vi "set_safe_mode.vi"(8 "error in (no error)":errorcluster, 10 "exit safe mode? (F)":bool, 11 "LightSourceMH110124MaiTai in":refnum<class "LightSourceMH110124MaiTai.lvclass">) -> (0 "error out":errorcluster, 3 "LightSourceMH110124MaiTai out":refnum<class "LightSourceMH110124MaiTai.lvclass">)   [LabVIEW 2010, in "LightSourceMH110124MaiTai.lvclass"]
uses:
  LightSourceMH110124MaiTai.lvclass
  LightSourceMH110124MaiTai.lvclass/LightSourceMH110124MaiTai.ctl
  class_data.vi
panel:
  out "finished?":bool
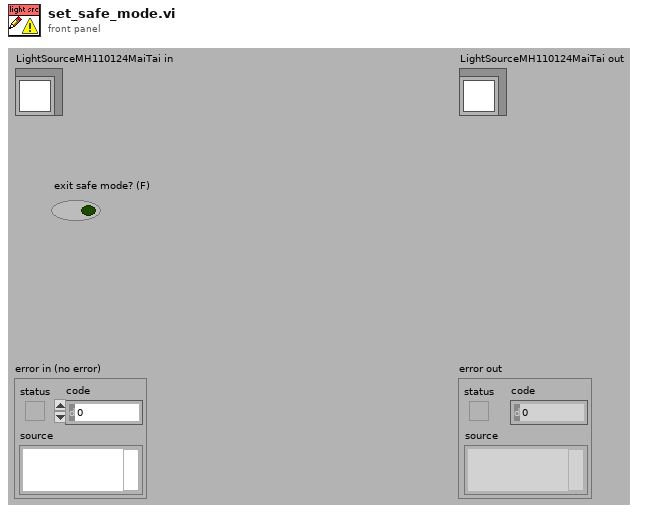
[diagram p1: front panel]
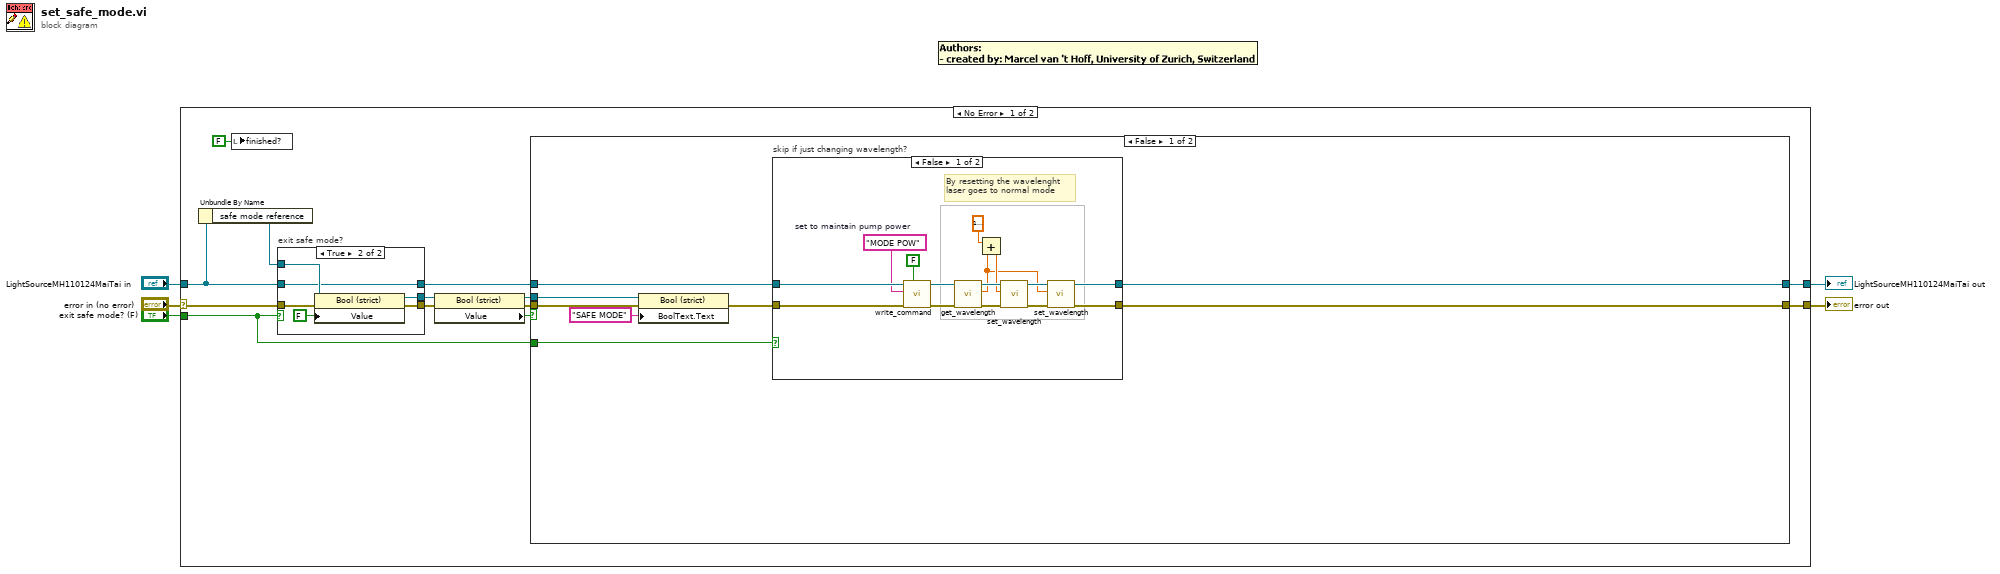
[diagram p0: block diagram]
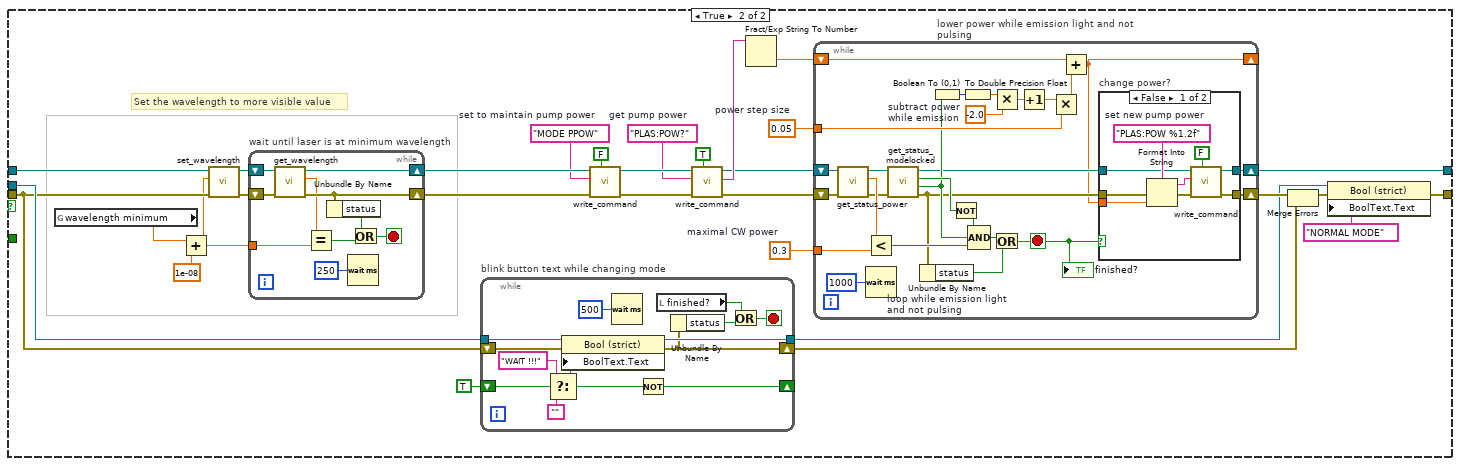
[diagram p4: hidden frame]
diagram:
  n1 = case shown="No Error" "error in (no error)" {
    selector: "error in (no error)" -> [w11 w145]
    tunnel: "LightSourceMH110124MaiTai in" -> [w7 w144]
    tunnel: [w14 w145] -> w3
    tunnel: [w13 w144] -> w2
    tunnel: "exit safe mode? (F)" -> [w6 _]
    frame No Error {
      n2 = Unbundle By Name(w7) -> ("safe mode reference"=w12:refnum<vi>)
      n3 = local write "finished?"(FALSE ("finished?")) -> ()
      n4 = case "exit safe mode?" shown="True" w6 {
        tunnel: w12 -> [w20 w27]
        tunnel: w11 -> [w21 w26]
        tunnel: [w21 w25] -> w10
        tunnel: [w20 w24] -> w9
        tunnel: [w19 w23] -> w8
        tunnel: w7 -> [w19 w23]
        frame False {
        }
        frame True {
          n5 = property class="Bool (strict)"(reference=w27, error in=w26, "Value"=FALSE) -> (reference out=w24:refnum<vi>, error out=w25:errorcluster)
        }
      }
      n6 = property class="Bool (strict)"(reference=w9, error in=w10) -> (reference out=w15:refnum<vi>, error out=w16:errorcluster, "Value"=w17:bool)
      n7 = case shown="False" w17 {
        tunnel: w16 -> [w33 w68]
        tunnel: w15 -> [w34 w70]
        tunnel: w8 -> [w32 w81]
        tunnel: [w30 w56] -> w14
        tunnel: [w29 w55] -> w13
        tunnel: w6 -> [w28 _]
        frame False {
          n8 = property class="Bool (strict)"(reference=w34, error in=w33, "BoolText.Text"="SAFE MODE" ("Boolean Text.Text")) -> (error out=w31:errorcluster)  [unwired: 1 out]
          n9 = case "skip if just changing wavelength?" shown="False" w28 {
            tunnel: w32 -> [w50 w52]
            tunnel: w31 -> [w43 w51]
            tunnel: [w37 w51] -> w30
            tunnel: [w36 w52] -> w29
            frame False {
              w41 = "MODE POW"  # set to maintain pump power
              # "By resetting the wavelenght\nlaser goes to normal mode"
              n10 = call-dynamic "write_command.vi"("read (T)"=FALSE, "error in (no error)"=w43, "string to write"=w41, "LightSourceMH110124MaiTai in"=w50) -> ("error out"=w46:errorcluster, "LightSourceMH110124MaiTai out"=w49:refnum<class "LightSourceMH110124MaiTai.lvclass">)  [unwired: 5 in, 1 out]
              n11 = call-dynamic "get_wavelength.vi"("error in (no error)"=w46, "LightSourceMH110124MaiTai in"=w49) -> ("error out"=w45:errorcluster, "wavelength"=w38:dbl[unit], "LightSourceMH110124MaiTai out"=w48:refnum<class "LightSourceMH110124MaiTai.lvclass">)  [unwired: 7 in]
              n12 = Add(x=dbl[unit] 1e-09 ("y"), y=w38) -> (x+y=w39:dbl[unit])
              n13 = call-dynamic "set_wavelength.vi"("error in (no error)"=w45, "wavelength in"=w39, "LightSourceMH110124MaiTai in"=w48) -> ("error out"=w44:errorcluster, "LightSourceMH110124MaiTai out"=w47:refnum<class "LightSourceMH110124MaiTai.lvclass">)  [unwired: 7 in]
              n14 = call-dynamic "set_wavelength.vi"("error in (no error)"=w44, "wavelength in"=w38, "LightSourceMH110124MaiTai in"=w47) -> ("error out"=w37:errorcluster, "LightSourceMH110124MaiTai out"=w36:refnum<class "LightSourceMH110124MaiTai.lvclass">)  [unwired: 7 in]
            }
            frame True {
            }
          }
        }
        frame True {
          w64 = dbl[unit] 0.3  # maximal CW power
          w63 = 0.05  # power step size
          w73 = "PLAS:POW?"  # get pump power
          w76 = "MODE PPOW"  # set to maintain pump power
          # "Set the wavelength to more visible value"
          n15 = global read "class_data.vi" "wavelength minimum"() -> (w53:dbl[unit])
          n16 = Add(x=w53, y=dbl[unit] 1e-08) -> (x+y=w54:dbl[unit])
          n17 = call-dynamic "set_wavelength.vi"("error in (no error)"=w68, "wavelength in"=w54, "LightSourceMH110124MaiTai in"=w81) -> ("error out"=w79:errorcluster, "LightSourceMH110124MaiTai out"=w80:refnum<class "LightSourceMH110124MaiTai.lvclass">)  [unwired: 7 in]
          n18 = while "wait until laser is at minimum wavelength" {
            tunnel: w54 -> [w135]
            shift-right: [w137] -> w77
            shift-left: w79 -> [w138]
            shift-right: [w134] -> w78
            shift-left: w80 -> [w139]
            stop <- w140 stop-if-true
            n19 = call-dynamic "get_wavelength.vi"("error in (no error)"=w138, "LightSourceMH110124MaiTai in"=w139) -> ("error out"=w137:errorcluster, "wavelength"=w136:dbl[unit], "LightSourceMH110124MaiTai out"=w134:refnum<class "LightSourceMH110124MaiTai.lvclass">)  [unwired: 7 in]
            n20 = Equal?(x=w136, y=w135) -> (x = y?=w142:bool)
            n21 = Unbundle By Name(w137) -> ("status"=w141:bool)
            n22 = Wait (ms)(milliseconds to wait=u32 250) -> ()  [unwired: 1 out]
            n23 = Or(x=w141, y=w142) -> (x .or. y?=w140:bool)
          }
          n24 = while "blink button text while changing mode" {
            tunnel: w70 -> [w133]
            tunnel: [w132] -> w59
            shift-right: [w121] -> _
            shift-left: TRUE -> [w124]
            shift-right: [w130] -> w60
            shift-left: w68 -> [w131]
            stop <- w129 stop-if-true
            n25 = Select(t="WAIT !!!" ("Boolean Text.Text"), s=w124, f="") -> (s? t:f=w126:string)
            n26 = property class="Bool (strict)"(reference=w133, error in=w131, "BoolText.Text"=w126) -> (reference out=w132:refnum<vi>, error out=w130:errorcluster)
            n27 = Wait (ms)(milliseconds to wait=u32 500) -> ()  [unwired: 1 out]
            n28 = Not(x=w124) -> (.not. x?=w121:bool)
            n29 = local read "finished?"() -> (w122:bool)
            n30 = Unbundle By Name(w130) -> ("status"=w123:bool)
            n31 = Or(x=w122, y=w123) -> (x .or. y?=w129:bool)
          }
          n32 = call-dynamic "write_command.vi"("read (T)"=FALSE, "error in (no error)"=w77, "string to write"=w76, "LightSourceMH110124MaiTai in"=w78) -> ("error out"=w74:errorcluster, "LightSourceMH110124MaiTai out"=w75:refnum<class "LightSourceMH110124MaiTai.lvclass">)  [unwired: 5 in, 1 out]
          n33 = call-dynamic "write_command.vi"("read (T)"=TRUE, "error in (no error)"=w74, "string to write"=w73, "LightSourceMH110124MaiTai in"=w75) -> ("error out"=w65:errorcluster, "read string"=w67:string, "LightSourceMH110124MaiTai out"=w66:refnum<class "LightSourceMH110124MaiTai.lvclass">)  [unwired: 5 in]
          n34 = Fract/Exp String To Number(string=w67) -> (number=w62:dbl)  [unwired: 3 in, 1 out]
          n35 = while "lower power while emission light and not pulsing" {
            shift-right: [w83] -> w61
            shift-left: w65 -> [w108]
            shift-right: [w84] -> w55
            shift-left: w66 -> [w109]
            tunnel: w64 -> [w106]
            tunnel: w63 -> [w97]
            shift-right: [w85] -> _
            shift-left: w62 -> [w89]
            stop <- w88 stop-if-true
            n36 = call-dynamic "get_status_power.vi"("error in (no error)"=w108, "LightSourceMH110124MaiTai in"=w109) -> ("error out"=w105:errorcluster, "output power"=w107:dbl[unit], "LightSourceMH110124MaiTai out"=w104:refnum<class "LightSourceMH110124MaiTai.lvclass">)  [unwired: 7 in]
            n37 = Less?(x=w107, y=w106) -> (x < y?=w91:bool)
            n38 = Wait (ms)(milliseconds to wait=u32 1000) -> ()  [unwired: 1 out]
            n39 = call-dynamic "get_status_modelocked.vi"("error in (no error)"=w105, "LightSourceMH110124MaiTai in"=w104) -> ("error out"=w86:errorcluster, "Emission"=w92:bool, "Pulsing"=w93:bool, "LightSourceMH110124MaiTai out"=w87:refnum<class "LightSourceMH110124MaiTai.lvclass">)  [unwired: 6 in]
            n40 = Unbundle By Name "loop while emission light\nand not pulsing"(w86) -> ("status"=w95:bool)
            n41 = Boolean To (0,1) "subtract power \nwhile emission"(Boolean=w92) -> (0, 1=w100:i16)
            n42 = Not(x=w93) -> (.not. x?=w94:bool)
            n43 = To Double Precision Float(number=w100) -> (double precision float=w101:dbl)
            n44 = Compound Arithmetic op=AND(w94, w92, w91) -> (w96:bool)
            n45 = Multiply(x=w101, y=-2.0) -> (x*y=w99:dbl)
            n46 = Or(x=w96, y=w95) -> (x .or. y?=w88:bool)
            "finished?" <- w88
            n47 = Increment(x=w99) -> (x+1=w102:dbl)
            n48 = Multiply(x=w102, y=w97) -> (x*y=w90:dbl)
            n49 = Add(x=w89, y=w90) -> (x+y=w85:dbl)
            n50 = case "change power?" shown="False" w88 {
              tunnel: w87 -> [w116 w120]
              tunnel: w86 -> [w114 w119]
              tunnel: w85 -> [w118 _]
              tunnel: [w111 w120] -> w84
              tunnel: [w110 w119] -> w83
              frame False {
                w117 = "PLAS:POW %1.2f"  # set new pump power
                n51 = Format Into String(format string=w117, error in=w114, w118) -> (resulting string=w115:string, error out=w113:errorcluster)  [unwired: 1 in]
                n52 = call-dynamic "write_command.vi"("read (T)"=FALSE, "error in (no error)"=w113, "string to write"=w115, "LightSourceMH110124MaiTai in"=w116) -> ("error out"=w110:errorcluster, "LightSourceMH110124MaiTai out"=w111:refnum<class "LightSourceMH110124MaiTai.lvclass">)  [unwired: 5 in, 1 out]
              }
              frame True {
              }
            }
          }
          n53 = Merge Errors(w61, w60) -> (w58:errorcluster)
          n54 = property class="Bool (strict)"(reference=w59, error in=w58, "BoolText.Text"="NORMAL MODE" ("Boolean Text.Text")) -> (error out=w56:errorcluster)  [unwired: 1 out]
        }
      }
    }
    frame Error {
    }
  }
  "error out" <- w3
  "LightSourceMH110124MaiTai out" <- w2
